vi "ReadCoins.vi"(8 "error in (no error)":errorcluster) -> (0 "error out":errorcluster, 3 "Value":cluster{"Numeric":dbl, "Boolean Text":string}[](array[cluster]))   [LabVIEW 2020, in "Coins.lvlib"]
uses:
  Coins.lvlib
  <vilib>/Utility/xml.llb/Read From XML File(string).vi
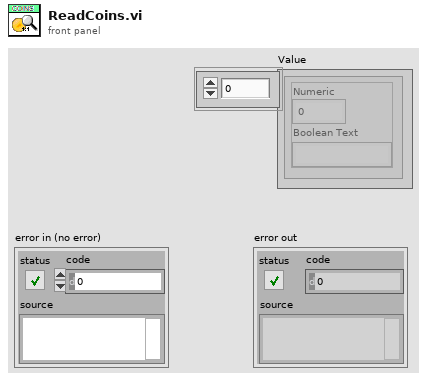
[diagram p1: front panel]
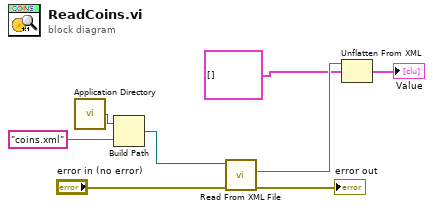
[diagram p0: block diagram]
diagram:
  n1 = call <vilib>:"Application Directory.vi"() -> ("Application Directory"=w7:path)
  n2 = Build Path(base path=w7, name or relative path="coins.xml") -> (appended path=w5:path)
  n3 = call-poly <vilib>:"Read From XML File.vi"("error in (no error)"="error in (no error)", "XML File Path"=w5) -> ("error out"=→"error out":errorcluster, "XML Elements"=w4:string)  [unwired: 7 in, 1 out]
  n4 = Unflatten From XML(xml string=w4, type=cluster{"Numeric":dbl, "Boolean Text":string}[] [] ("Value")) -> (value=→"Value":cluster{"Numeric":dbl, "Boolean Text":string}[])  [unwired: 1 in, 1 out]
